vi "Lissajous Patterns.vi"() -> ()   [LabVIEW 2025]
uses:
  <vilib>/numeric/Random Number (Range) U64.vi
  <vilib>/numeric/sub_Random U32.vi
panel:
  in  "stop":bool
  out "XY Graph":cluster{"Y":dbl[], "Y":dbl[]}[](graph)
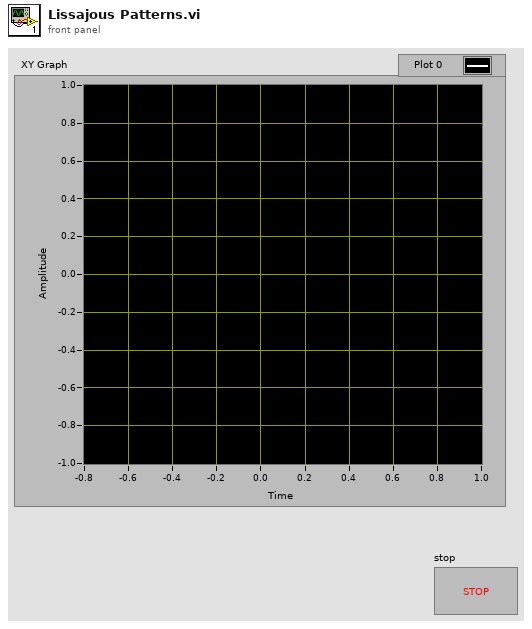
[diagram p1: front panel]
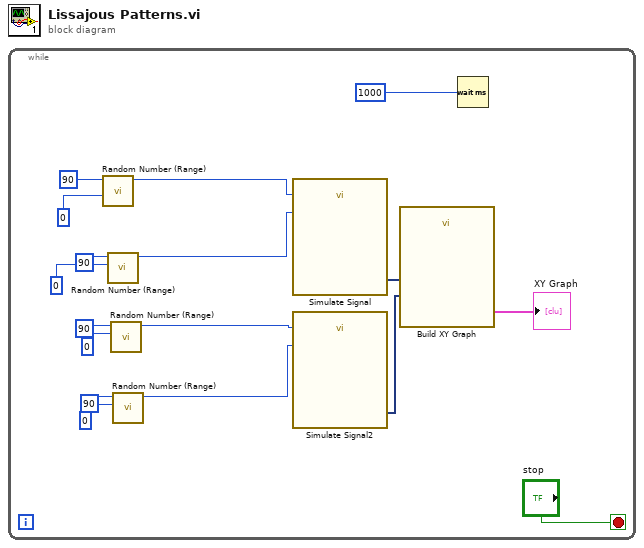
[diagram p0: block diagram]
diagram:
  n1 = while {
    stop <- "stop" stop-if-true
    n2 = call-poly <vilib>:"Random Number (Range).vi"("lower bound (0)"=u64 0, "upper bound (100)"=u64 90) -> ("number"=w12:u64)  [unwired: 9 in]
    n3 = call-poly <vilib>:"Random Number (Range).vi"("lower bound (0)"=u64 0, "upper bound (100)"=u64 90) -> ("number"=w5:u64)  [unwired: 9 in]
    n4 = call-poly <vilib>:"Random Number (Range).vi"("lower bound (0)"=u64 0, "upper bound (100)"=u64 90) -> ("number"=w4:u64)  [unwired: 9 in]
    n5 = call-poly <vilib>:"Random Number (Range).vi"("lower bound (0)"=u64 0, "upper bound (100)"=u64 90) -> ("number"=w3:u64)  [unwired: 9 in]
    n6 = call "Simulate Signal"("Frequency"=w12, "Phase"=w5) -> ("Sine"=w16:dynamicdata)  [unwired: 12 in, 1 out]
    n7 = call "Simulate Signal2"("Frequency"=w4, "Phase"=w3) -> ("Sine"=w15:dynamicdata)  [unwired: 12 in, 1 out]
    n8 = call "Build XY Graph"("Y Input"=w15, "X Input"=w16) -> ("XY Graph"=→"XY Graph":cluster{"X":dbl[], "Y":dbl[]}[])  [unwired: 8 in, 1 out]
    n9 = Wait (ms)(milliseconds to wait=u32 1000) -> ()  [unwired: 1 out]
  }
